vi "Remove Section.vi"(7 "Section":string, 8 "error in (no error)":errorcluster, 11 "Ini Path in":path) -> (0 "error out":errorcluster, 2 "Section Found?":bool, 3 "Ini Path out":path)   [LabVIEW 2018, in "Config.lvlib"]
uses:
  Config.lvlib
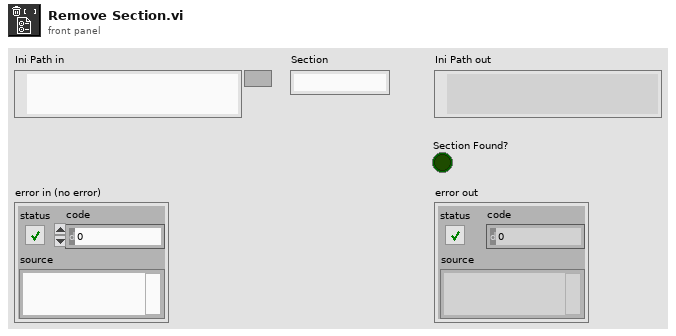
[diagram p1: front panel]
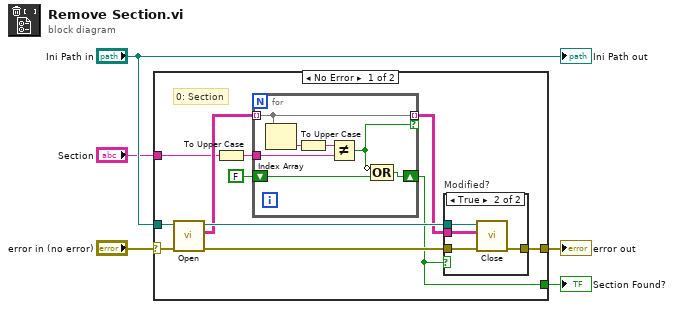
[diagram p0: block diagram]
diagram:
  n1 = case shown="No Error" "error in (no error)" {
    selector: "error in (no error)" -> [w16 w29]
    tunnel: [w15 w29] -> w1
    tunnel: "Ini Path in" -> [w13 _]
    tunnel: "Section" -> [w8 _]
    tunnel: [w6 _] -> w2
    frame No Error {
      # "0: Section"
      n2 = call "Open.vi"("error in (no error)"=w16, "Ini Path in"=w13) -> ("error out"=w12:errorcluster, "skvc out"=w9:string[][], "Ini Path out"=w14:path)  [unwired: 6 in, 1 out]
      n3 = To Upper Case(1:w8) -> (0:w11:string)
      n4 = for {
        tunnel: w9 -> [w25] mode=indexing
        tunnel: w11 -> [w26]
        tunnel: [w25] -> w7 mode=indexing if=w24
        shift-right: [w22] -> w6
        shift-left: FALSE -> [w23]
        n5 = Index Array(array=w25) -> (element=w28:string)  [unwired: 1 in]
        n6 = To Upper Case(1:w28) -> (0:w27:string)
        n7 = Not Equal?(x=w27, y=w26) -> (x != y?=w24:bool)
        n8 = Compound Arithmetic op=OR(invert w24, w23) -> (w22:bool)
      }
      n9 = case "Modified?" shown="True" w6 {
        tunnel: w12 -> [w17 w21]
        tunnel: [w17 w20] -> w15
        tunnel: w14 -> [_ w19]
        tunnel: w7 -> [_ w18]
        frame False {
        }
        frame True {
          n10 = call "Close.vi"("error in (no error)"=w21, "skvc in"=w18, "Ini Path in"=w19) -> ("error out"=w20:errorcluster)  [unwired: 7 in, 1 out]
        }
      }
    }
    frame Error {
    }
  }
  "error out" <- w1
  "Section Found?" <- w2
  "Ini Path out" <- "Ini Path in"
